vi "Range.vi"(8 "error in (no error)":errorcluster, 9 "length":i32, 10 "index":i32, 11 "[V] Main UI in":refnum<class "[V] Main UI.lvclass">) -> (0 "error out":errorcluster, 3 "[V] Main UI out":refnum<class "[V] Main UI.lvclass">)   [LabVIEW 2020, in "[V] Main UI.lvlib" / "[V] Main UI.lvclass"]
uses:
  [V] Main UI.lvclass
  MVVM Framework/MVVM Abstruct View/MVVM Abstruct View/MVVM Abstruct View.lvclass/MVVM Abstruct View.ctl
  Models/Data Loader/Data Load Interface/Data Load Interface Messages/File Range Msg/File Range Msg.lvclass/File Range Msg.ctl
  <vilib>/ActorFramework/Message Enqueuer/Message Enqueuer.lvclass/Message Enqueuer.ctl
  MVVM Framework/MVVM Abstruct View/MVVM Abstruct View/Accessor/Read ActorMap-Models.vi
  <vilib>/ActorFramework/Message Enqueuer/Enqueue.vi
  Models/Data Loader/Data Load Interface/Data Load Interface Messages/File Range Msg/File Range Msg.lvclass
  C:/Program Files (x86)/National Instruments/LabVIEW 2020/vi.lib/ActorFramework/Message/Message.lvclass
  <vilib>/ActorFramework/Message Priority Queue/Priority Enqueue.vi
  Depden On/ActorMap/ActorMap.lvclass
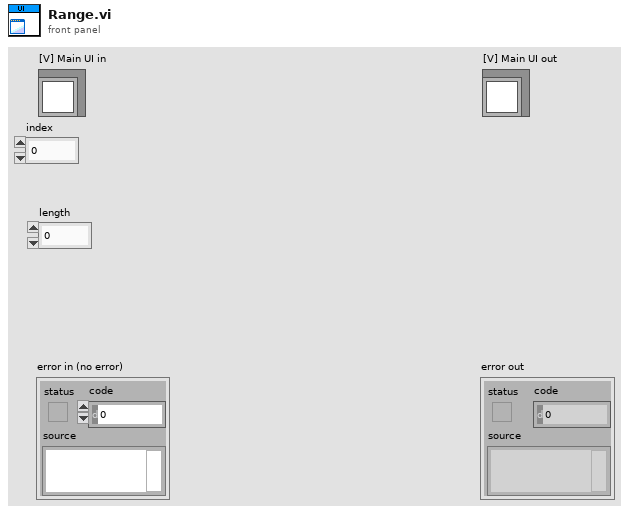
[diagram p1: front panel]
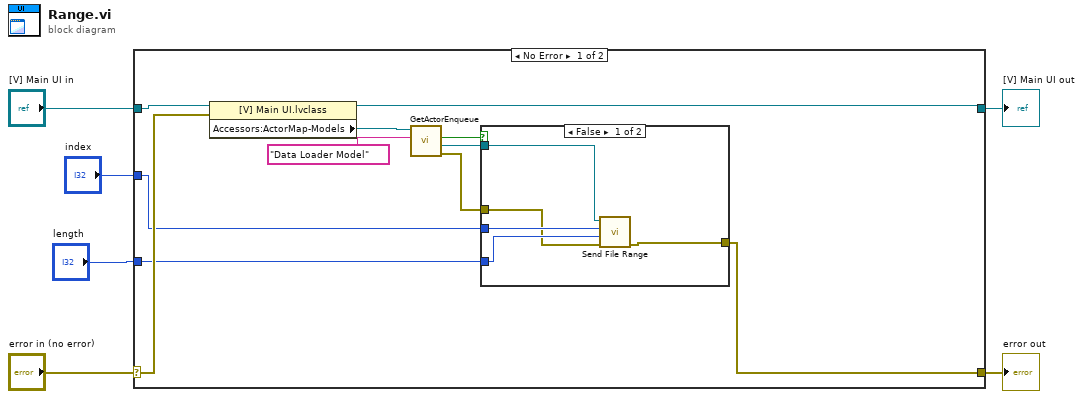
[diagram p0: block diagram]
diagram:
  n1 = case shown="No Error" "error in (no error)" {
    selector: "error in (no error)" -> [w11 w25]
    tunnel: [w7 w25] -> w5
    tunnel: [w10 w24] -> w3
    tunnel: "[V] Main UI in" -> [w12 w24]
    tunnel: "index" -> [w9 _]
    tunnel: "length" -> [w8 _]
    frame No Error {
      n2 = property class="[V] Main UI.lvclass"(reference=w12, error in=w11) -> (reference out=w10:refnum<class "[V] Main UI.lvclass">, "Accessors:ActorMap-Models"=w17:refnum<class "ActorMap.lvclass">)  [unwired: 1 out]
      n3 = call "GetActorEnqueue.vi"("name"="Data Loader Model", "ActorMap in"=w17) -> ("error out"=w13:errorcluster, "Enqueue"=w14:refnum<class "Message Enqueuer.lvclass">, "key not found?"=w15:bool)  [unwired: 6 in, 1 out]
      n4 = case shown="False" w15 {
        tunnel: w14 -> [w22 _]
        tunnel: w13 -> [w19 w23]
        tunnel: [w18 w23] -> w7
        tunnel: w9 -> [w21 _]
        tunnel: w8 -> [w20 _]
        frame False {
          n5 = call "Send File Range.vi"("error in (no error)"=w19, "End(%)"=w20, "start(%)"=w21, "Message Enqueuer"=w22) -> ("error out"=w18:errorcluster)  [unwired: 6 in, 1 out]
        }
        frame True {
        }
      }
    }
    frame Error {
    }
  }
  "error out" <- w5
  "[V] Main UI out" <- w3
